vi "Stop Core.vi"(10 "final error code":i32, 11 "CameraTestingUI in":refnum<class "CameraTestingUI.lvclass">) -> (3 "CameraTestingUI out":refnum<class "CameraTestingUI.lvclass">)   [LabVIEW 2020, in "CameraTestingUI.lvlib" / "CameraTestingUI.lvclass"]
doc: "(<B>Filename</B>: Actor Framework.lvlib:Actor.lvclass:Stop Core.vi)\n\nDefines what the actor does before it stops. Use the <B>final error code</B> input to determine whether the actor shut down in response to an error.\n\nBy default, this method passes the Stop message along to all auto-stop nested actors. A descendant class may override this method to define additional behavior, such as shutting down any processes the actor initiated in its override of the Actor Core method."
uses:
  CameraTestingUI.lvclass
  <vilib>/ActorFramework/Actor/Actor.lvclass
  CameraTestingUI.lvclass/CameraTestingUI.ctl
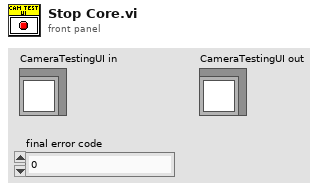
[diagram p1: front panel]
types:
  T1 = typedef "CameraTestingUI.lvlib/CameraTestingUI.lvclass/QuitActorEvn.ctl" = refnum<user-event>
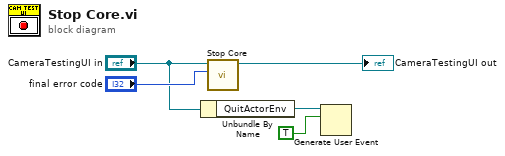
[diagram p0: block diagram]
diagram:
  n1 = Unbundle By Name("CameraTestingUI in") -> ("QuitActorEnv"=w2:T1)
  n2 = call-parent "Stop Core.vi"("final error code"="final error code", "Actor in"="CameraTestingUI in") -> ("Actor out"=→"CameraTestingUI out":refnum<class "CameraTestingUI.lvclass">)  [unwired: 9 in]
  n3 = Generate User Event(user event=w2, event data cluster=TRUE ("event data")) -> ()  [unwired: 2 in, 2 out]
